vi "Read 1D Array SGL.vi"(8 "error in (no error)":errorcluster, 9 "start index (0)":i64, 10 "number of elements":i64, 11 "pointer in":u64) -> (0 "error out":errorcluster, 1 "start index out":i64, 2 "value":sgl[](array[numeric]), 3 "pointer out":u64)   [LabVIEW 2013, in "Linux RT IPC.Shared Memory.lvlib"]
uses:
  Linux RT IPC.Shared Memory.lvlib
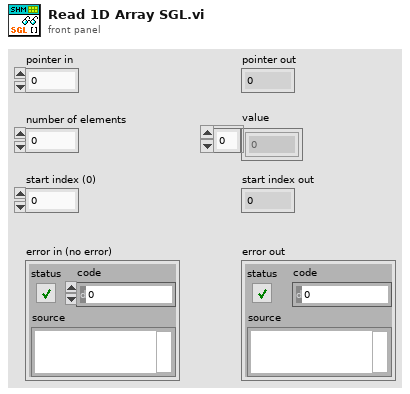
[diagram p1: front panel]
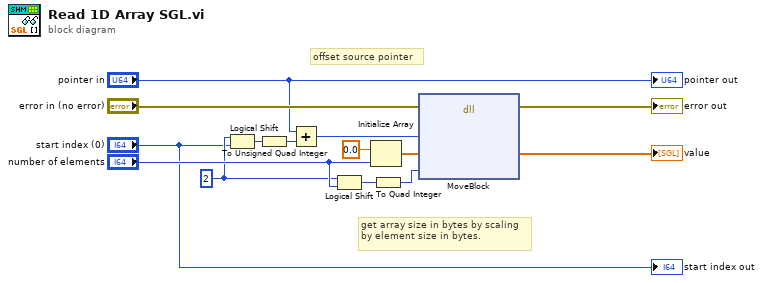
[diagram p0: block diagram]
diagram:
  w2 = i16 2 ("y")
  # "get array size in bytes by scaling by element size in bytes."
  # "offset source pointer"
  n1 = Logical Shift(y=w2, x="start index (0)") -> (x << y=w8:i64)
  n2 = To Unsigned Quad Integer(1:w8) -> (0:w7:u64)
  n3 = Add(x="pointer in", y=w7) -> (x+y=w3:u64)
  n4 = Logical Shift(y=w2, x="number of elements") -> (x << y=w9:i64)
  n5 = Initialize Array(sgl 0.0, "number of elements") -> (w5:sgl[])
  n6 = To Quad Integer(1:w9) -> (0:w4:i64)
  n7 = dll-call lib="LabVIEW" fn="MoveBlock"(error in="error in (no error)", "pointer"=w3, "data"=w5, "size"=w4) -> (error out=→"error out":errorcluster, "data"=→"value":sgl[])  [unwired: 5 in, 1 out]
  "pointer out" <- "pointer in"
  "start index out" <- "start index (0)"
